vi "Measurement.vi"(8 "Fehler (Eingang\n, kein Fehler)":errorcluster caption="Fehler (Eingang, kein Fehler)") -> (0 "Fehler (Ausgang)":errorcluster)   [LabVIEW 2020]
uses:
  <vilib>/DAQmx/read.llb/DAQmx Read (Counter DBL 1Chan 1Samp).vi
  <vilib>/DAQmx/read.llb/DAQmx Read (Counter U32 1Chan 1Samp).vi
  <vilib>/DAQmx/miscellaneous.llb/DAQmx Fill In Error Info.vi
  <vilib>/DAQmx/create/channels.llb/DAQmx Create Channel (CI-Count Edges).vi
  <vilib>/ptbypt/NI_PtbyPt.lvlib
  <resource>/objmgr/daqmx.rc
panel:
  in  "Edge?":bool
  in  "stop":bool
  out "edge":u32
  in  "error in":errorcluster
  out "frequence":dbl format="%0.2f"
  in  "radius":dbl
  in  "counts Per Revolution":dbl=2048.0
  out "velocity":dbl
  out "Waveform Chart 2":dbl[](graph)
  out "largest Velocity":dbl
  in  "sampling point":i32=500
  out "trigger":bool
  in  "Record start value":dbl=100.0
  out "Waveform Chart":dbl(graph)
  out "Filename Out":path
  out "Saving Data":bool
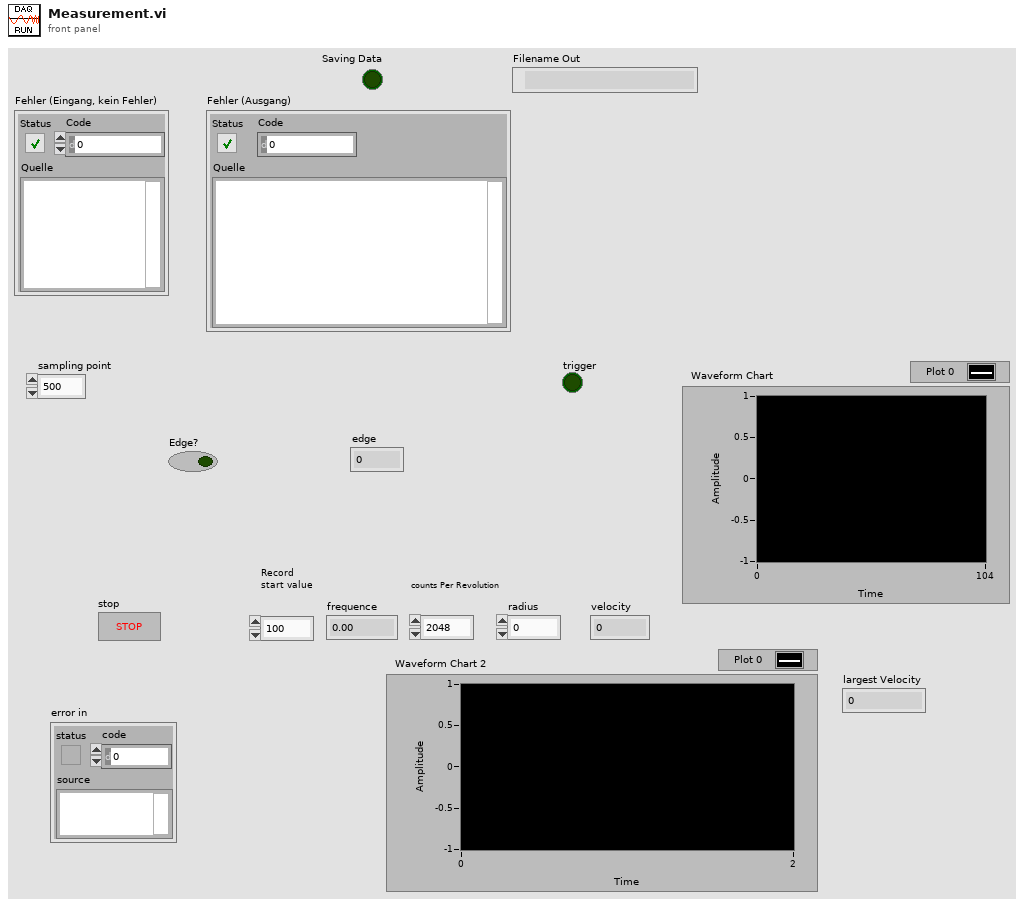
[diagram p1: front panel]
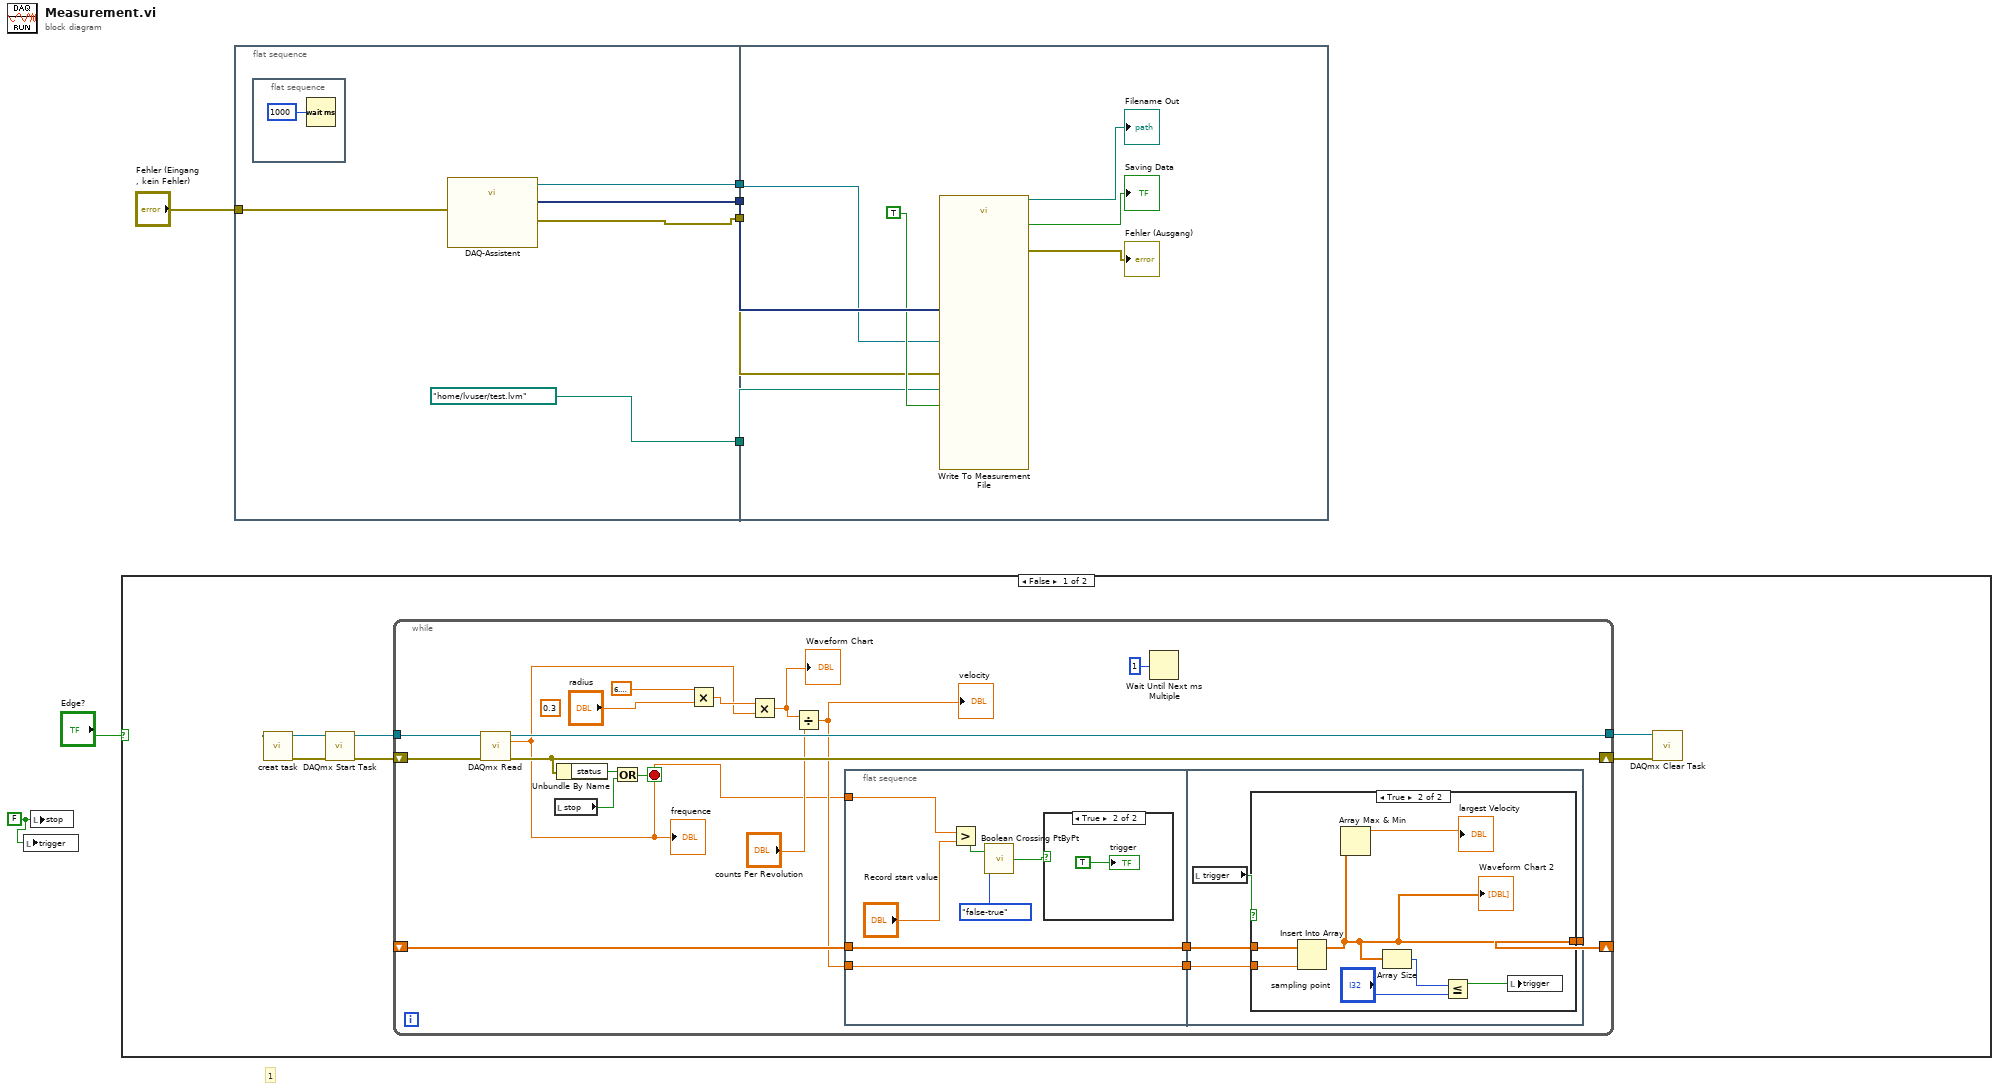
[diagram p0: block diagram]
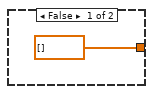
[diagram p3: hidden frame]
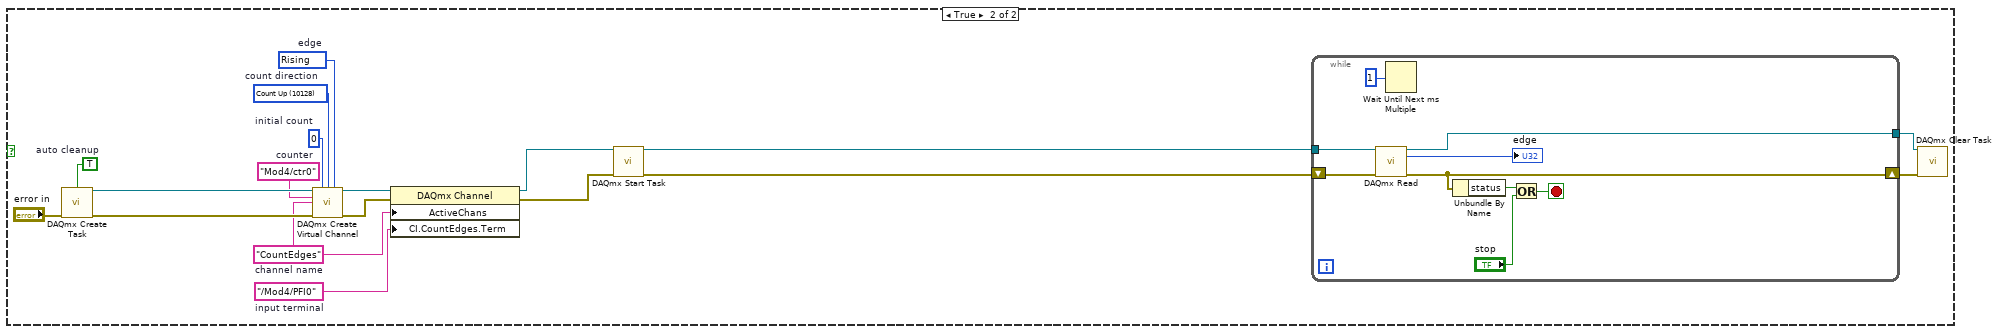
[diagram p4: hidden frame]
diagram:
  w1 = FALSE ("stop")
  # "1"
  n1 = local write "trigger"(w1) -> ()
  n2 = local write "stop"(w1) -> ()
  n3 = case shown="False" "Edge?" {
    frame False {
      n4 = call "creat task.vi"() -> ("error out"=w13:errorcluster, "task out"=w12:refnum<k21>)  [unwired: 10 in]
      n5 = call <vilib>:"DAQmx Start Task.vi"("task/channels in"=w12, "error in"=w13) -> ("task out"=w8:refnum<k21>, "error out"=w9:errorcluster)  [unwired: 12 in]
      n6 = while {
        tunnel: w8 -> [w32]
        tunnel: [w30] -> w11
        shift-right: [w29] -> w10
        shift-left: w9 -> [w31]
        shift-right: [w21] -> _
        shift-left: _ -> [w20]
        stop <- w27 stop-if-true
        (unwired) 0.3 ("radius")
        n7 = call-poly <vilib>:"DAQmx Read.vi"("task/channels in"=w32, "error in"=w31) -> ("task out"=w30:refnum<k21>, "data"=w15:dbl, "error out"=w29:errorcluster)  [unwired: 11 in]
        "frequence" <- w15
        n8 = local read "stop"() -> (w22:bool)
        n9 = Unbundle By Name(w29) -> ("status"=w28:bool)
        n10 = Or(x=w28, y=w22) -> (x .or. y?=w27:bool)
        n11 = Multiply(x=6.283185307179586, y="radius") -> (x*y=w24:dbl)
        n12 = Multiply(x=w24, y=w15) -> (x*y=w16:dbl)
        "Waveform Chart" <- w16
        n13 = Divide(x=w16, y="counts Per Revolution") -> (x/y=w17:dbl)
        "velocity" <- w17
        n14 = flat-sequence {
          tunnel: w20 -> [w38]
          tunnel: w17 -> [w39]
          tunnel: [w39] -> w19
          tunnel: [w38] -> w18
          tunnel: w15 -> [w35]
          tunnel: [w43] -> w21
          tunnel: w19 -> [w44]
          tunnel: w18 -> [w42]
          frame #0 {
            n15 = Greater?(x=w35, y="Record start value") -> (0:w36:bool)
            n16 = call <vilib>:"Boolean Crossing PtByPt.vi"("direction"=enum16{"either", "false-true", "true-false"}."false-true", "input"=w36) -> ("crossing"=w34:bool)  [unwired: 1 in]
            n17 = case shown="True" w34 {
              frame False {
              }
              frame True {
                "trigger" <- TRUE ("x >= y?")
              }
            }
          }
          frame #1 {
            n18 = local read "trigger"() -> (w41:bool)
            n19 = case shown="True" w41 {
              tunnel: w44 -> [_ w52]
              tunnel: [dbl[] [] w48] -> w43
              tunnel: w42 -> [_ w51]
              frame False {
              }
              frame True {
                n20 = Insert Into Array(array=w51, new element=w52) -> (w48:dbl[])  [unwired: 1 in]
                "Waveform Chart 2" <- w48
                n21 = Array Max & Min(array=w48) -> (max value=→"largest Velocity":dbl)  [unwired: 3 out]
                n22 = Array Size(array=w48) -> (size(s)=w50:i32)
                n23 = Less Or Equal?(x=w50, y="sampling point") -> (x <= y?=w46:bool)
                n24 = local write "trigger"(w46) -> ()
              }
            }
          }
        }
        n25 = Wait Until Next ms Multiple(millisecond multiple=u32 1) -> ()  [unwired: 1 out]
      }
      n26 = call <vilib>:"DAQmx Clear Task.vi"("task in"=w11, "error in"=w10) -> ()  [unwired: 13 in, 1 out]
    }
    frame True {
      w55 = "/Mod4/PFI0"  # input terminal
      w58 = 10280 items=["Rising"=10280, "Falling"=10171]  # edge
      w59 = 10128 items=["Count Up"=10128, "Count Down"=10124, "Externally Controlled"=10326]  # count direction
      w60 = u32 0  # initial count
      w56 = "CountEdges"  # channel name
      w62 = "Mod4/ctr0"  # counter
      w64 = TRUE  # auto cleanup
      n27 = call <vilib>:"DAQmx Create Task.vi"("auto cleanup"=w64, "error in"="error in") -> ("task out"=w63:refnum<k21>, "error out"=w65:errorcluster)  [unwired: 12 in]
      n28 = call-poly <vilib>:"DAQmx Create Virtual Channel.vi"("task in"=w63, "initial count"=w60, "count direction"=w59, "edge"=w58, "counter"=w62, "name to assign"=w56, "error in"=w65) -> ("task out"=w57:refnum<k21>, "error out"=w61:errorcluster)  [unwired: 7 in]
      n29 = property class="DAQmx Channel"(reference=w57, error in=w61, "ActiveChans"=w56, "CI.CountEdges.Term"=w55) -> (reference out=w54:refnum<k21>, error out=w53:errorcluster)
      n30 = call <vilib>:"DAQmx Start Task.vi"("task/channels in"=w54, "error in"=w53) -> ("task out"=w70:refnum<k21>, "error out"=w69:errorcluster)  [unwired: 12 in]
      n31 = while {
        tunnel: w70 -> [w79]
        tunnel: [w77] -> w67
        shift-right: [w75] -> w68
        shift-left: w69 -> [w78]
        stop <- w73 stop-if-true
        n32 = call-poly <vilib>:"DAQmx Read.vi"("task/channels in"=w79, "error in"=w78) -> ("task out"=w77:refnum<k21>, "data"=→"edge":u32, "error out"=w75:errorcluster)  [unwired: 11 in]
        n33 = Wait Until Next ms Multiple(millisecond multiple=u32 1) -> ()  [unwired: 1 out]
        n34 = Unbundle By Name(w75) -> ("status"=w76:bool)
        n35 = Or(x=w76, y="stop") -> (x .or. y?=w73:bool)
      }
      n36 = call <vilib>:"DAQmx Clear Task.vi"("task in"=w67, "error in"=w68) -> ()  [unwired: 13 in, 1 out]
    }
  }
  n37 = flat-sequence {
    tunnel: "Fehler (Eingang\n, kein Fehler)" -> [w84]
    tunnel: [w83] -> w6
    tunnel: [w82] -> w5
    tunnel: [path "/home/lvuser/test.lvm" ("Filename")] -> w4
    tunnel: [w81] -> w3
    tunnel: w6 -> [w90]
    tunnel: w5 -> [w86]
    tunnel: w4 -> [w87]
    tunnel: w3 -> [w88]
    frame #0 {
      n38 = flat-sequence {
        frame #0 {
          n39 = Wait (ms)(milliseconds to wait=u32 1000) -> ()  [unwired: 1 out]
        }
      }
      n40 = call "DAQ-Assistent"("error in"=w84) -> ("task out"=w82:refnum<k21>, "data"=w83:dynamicdata, "error out"=w81:errorcluster)  [unwired: 16 in]
    }
    frame #1 {
      n41 = call "Write To Measurement File"("Signals"=w90, "Reset"=TRUE, "error in (no error)"=w88, "Filename"=w87, "DAQmx Task"=w86) -> ("Filename Out"=→"Filename Out":path, "Saving Data"=→"Saving Data":bool, "error out"=→"Fehler (Ausgang)":errorcluster)  [unwired: 12 in]
    }
  }
